vi "LPT Heuristic Solution.vi"(8 "error in (no error)":errorcluster, 10 "Array":i32[](array[numeric]), 11 "OSSP_Problem in":refnum<class "OSSP_Problem.lvclass">) -> (0 "error out":errorcluster, 3 "LPT List Heuristic Solution":u16[](array[numeric]))   [LabVIEW 2013, in "GA.lvclass"]
uses:
  GA.lvclass
  OSSP_Problem.lvclass
  OSSP_Problem.lvclass/OSSP_Problem.ctl
  Scheduler_Class/Operation to Machine Job Tuple.vi
  Scheduler.lvclass
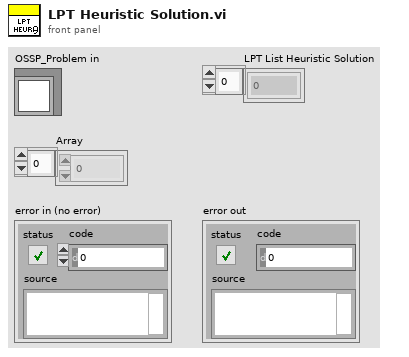
[diagram p1: front panel]
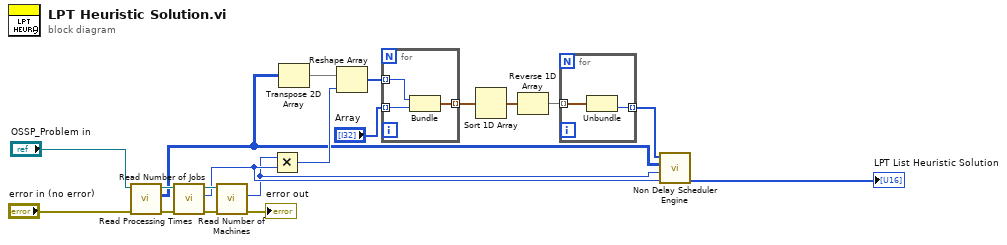
[diagram p0: block diagram]
diagram:
  n1 = call "Read Processing Times.vi"("error in (no error)"="error in (no error)", "OSSP_Problem in"="OSSP_Problem in") -> ("error out"=w10:errorcluster, "Processing Times"=w1:u16[][], "OSSP_Problem out"=w13:refnum<class "OSSP_Problem.lvclass">)  [unwired: 7 in]
  n2 = call "Read Number of Jobs.vi"("error in (no error)"=w10, "OSSP_Problem in"=w13) -> ("error out"=w11:errorcluster, "Number of Jobs"=w3:i32, "OSSP_Problem out"=w12:refnum<class "OSSP_Problem.lvclass">)  [unwired: 7 in]
  n3 = call "Read Number of Machines.vi"("error in (no error)"=w11, "OSSP_Problem in"=w12) -> ("error out"=→"error out":errorcluster, "Number of Machines"=w2:i32)  [unwired: 7 in, 1 out]
  n4 = Multiply(x=w2, y=w3) -> (x*y=w9:i32)
  n5 = Transpose 2D Array(2D array=w1) -> (transposed array=w14:u16[][])
  n6 = Reshape Array(w14, w9) -> (w8:u16[])
  n7 = for {
    tunnel: "Array" -> [w22] mode=indexing
    tunnel: w8 -> [w21] mode=indexing
    tunnel: [w20] -> w7 mode=indexing
    n8 = Bundle("Numeric"=w21, w22) -> (w20:cluster{"Numeric":u16, i32})  [unwired: 1 in]
  }
  n9 = Sort 1D Array(array=w7) -> (sorted array=w6:cluster{"Numeric":u16, i32}[])
  n10 = Reverse 1D Array(array=w6) -> (reversed array=w5:cluster{"Numeric":u16, i32}[])
  n11 = for {
    tunnel: w5 -> [w24] mode=indexing
    tunnel: [w23] -> w4 mode=indexing
    n12 = Unbundle(w24) -> (w23:i32)  [unwired: 1 out]
  }
  n13 = call "Non Delay Scheduler Engine.vi"("Number of  Jobs"=w3, "Number of Machines"=w2, "Processing Times"=w1, "Schedule"=w4) -> ("Reordered Schedule"=→"LPT List Heuristic Solution":u16[])  [unwired: 2 in, 5 out]
